vi "Read Loop.vi"(7 "Enum - Menu":enum16{"INIT", "READ", "RE-INIT", "CLOSE"}(ring), 8 "error in (no error)":errorcluster) -> (0 "error out":errorcluster, 1 "Isolated Gain":u32, 2 "DAQ Status":u32, 3 "Downlink Packet":T1)   [LabVIEW 2025]
panel:
  out "error out 2":errorcluster
  out "connection ID":refnum<k16>
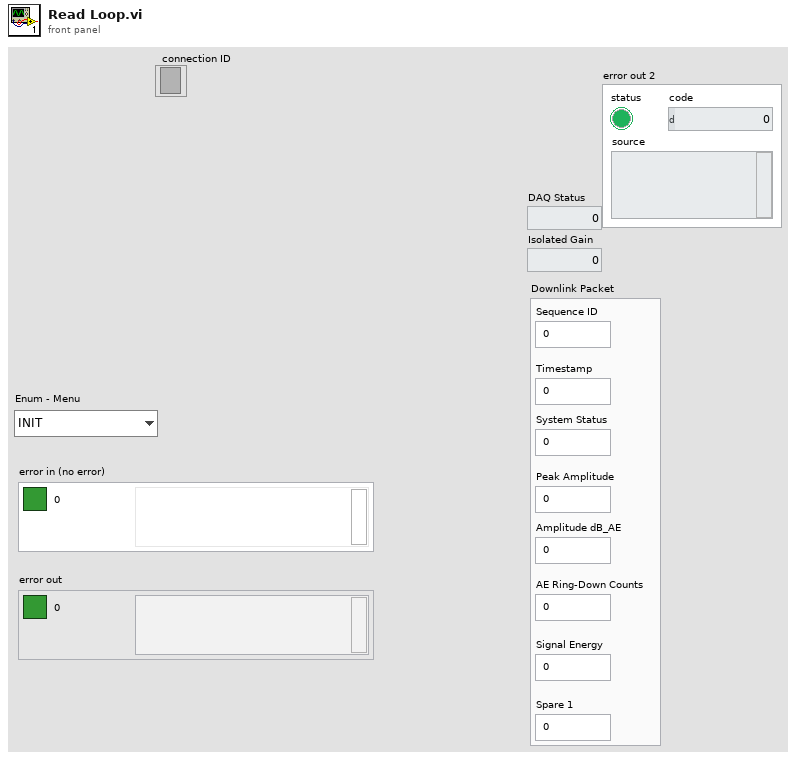
[diagram p1: front panel]
types:
  T1 = cluster{"Sequence ID":u32, "Timestamp":u32, "System Status":u32, "Peak Amplitude":u32, "Amplitude dB_AE":u32, "AE Ring-Down Counts":u32, "Signal Energy":u32, "Spare 1":u32}
  T2 = enum16{"big-endian, network order", "native, host order", "little-endian"}
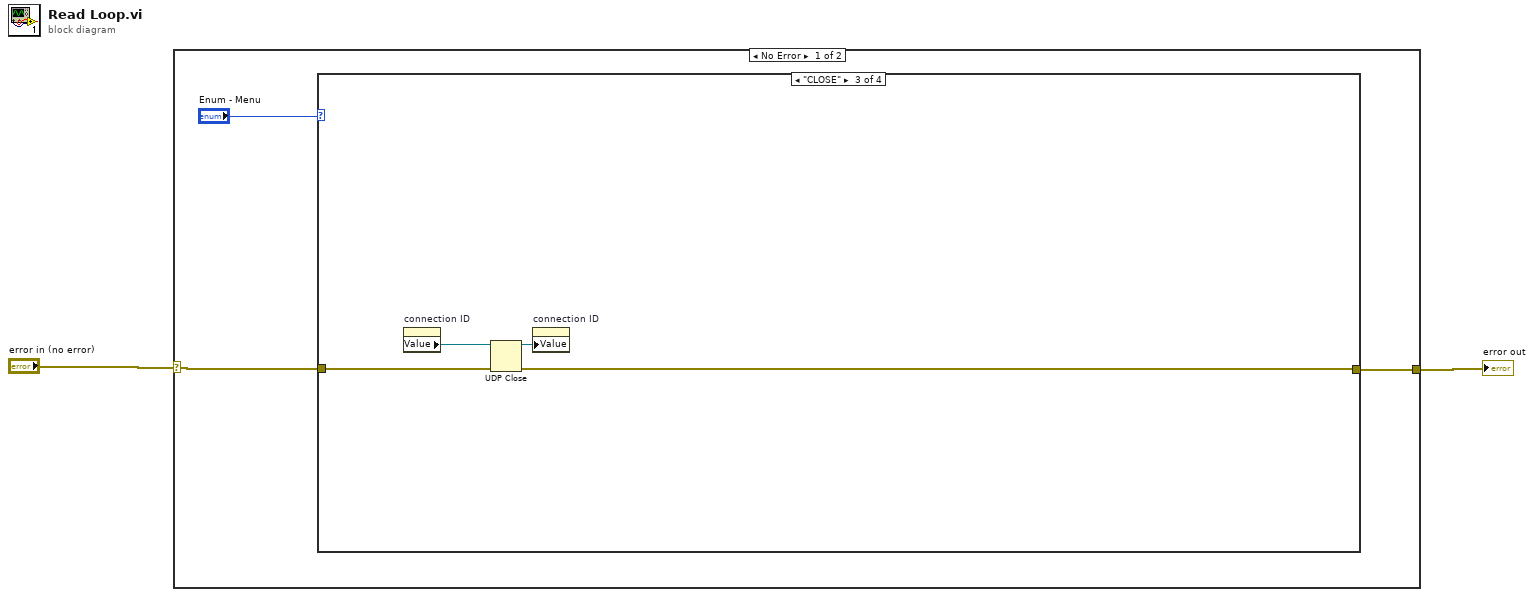
[diagram p0: block diagram]
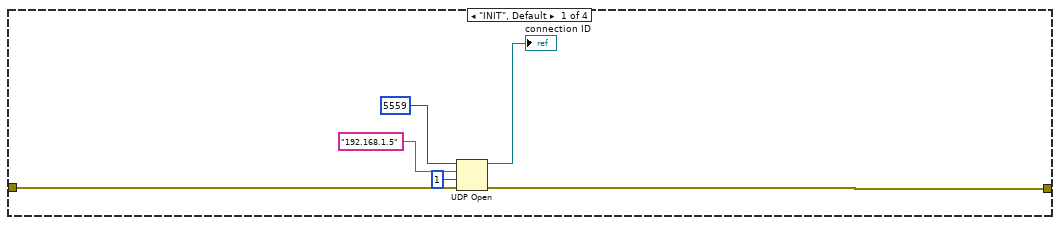
[diagram p2: hidden frame]
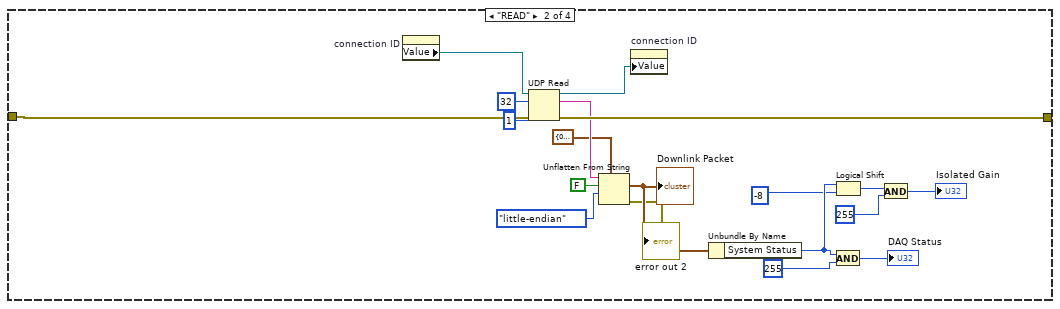
[diagram p3: hidden frame]
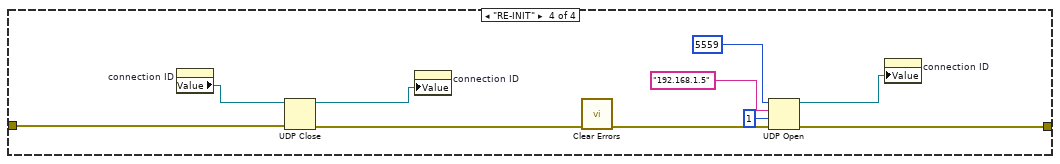
[diagram p4: hidden frame]
diagram:
  n1 = case shown="No Error" "error in (no error)" {
    selector: "error in (no error)" -> [w4 _]
    tunnel: [w3 _] -> w1
    frame No Error {
      n2 = case shown="\"CLOSE\"" "Enum - Menu" {
        tunnel: w4 -> [w10 w30 w32 w44]
        tunnel: [w9 w29 w31 w38] -> w3
        frame "INIT", Default {
          n3 = UDP Open(8:w10, 9:1 ("timeout ms (25000)"), 10:"192.168.1.5" ("service name"), 11:u16 5559 ("port")) -> (port=→"connection ID":refnum<k16>, 0:w9:errorcluster)  [unwired: 1 in, 1 out]
        }
        frame "READ" {
          n4 = property on="connection ID" class="Ref (strict)"() -> ("Value"=w27:refnum<k16>)  [unwired: 2 in, 2 out]
          n5 = UDP Read(connection ID=w27, max size (548)=32, timeout ms (25000)=1, 8:w30) -> (data out=w22:string, error out=w29:errorcluster, 3:w28:refnum<k16>)  [unwired: 2 out]
          n6 = Unflatten From String(type=T1 {"Sequence ID"=0, "Timestamp"=0, "System Status"=0, "Peak Amplitude"=0, "Amplitude dB_AE"=0, "AE Ring-Down Counts"=0, "Signal Energy"=0, "Spare 1"=0} ("Downlink Packet"), binary string=w22, data includes array or string size? (T)=FALSE ("prepend array or string size? (T)"), byte order (0:big-endian, network order)=T2."little-endian") -> (value=w20:T1, error out=→"error out 2":errorcluster)  [unwired: 1 in, 1 out]
          "Downlink Packet" <- w20
          n7 = property on="connection ID" class="Ref (strict)"("Value"=w28) -> ()  [unwired: 2 in, 2 out]
          n8 = Unbundle By Name(w20) -> ("System Status"=w17:u32)
          n9 = Logical Shift(y=w17, x=-8) -> (x << y=w15:i32)
          n10 = And(x=w17, y=u32 255) -> (x .and. y?=→"DAQ Status":u32)
          n11 = And(x=w15, y=u32 255) -> (x .and. y?=→"Isolated Gain":u32)
        }
        frame "CLOSE" {
          n12 = property on="connection ID" class="Ref (strict)"() -> ("Value"=w34:refnum<k16>)  [unwired: 2 in, 2 out]
          n13 = UDP Close(connection ID=w34, 8:w32) -> (connection ID out=w33:refnum<k16>, error out=w31:errorcluster)
          n14 = property on="connection ID" class="Ref (strict)"("Value"=w33) -> ()  [unwired: 2 in, 2 out]
        }
        frame "RE-INIT" {
          n15 = property on="connection ID" class="Ref (strict)"() -> ("Value"=w43:refnum<k16>)  [unwired: 2 in, 2 out]
          n16 = UDP Close(connection ID=w43, 8:w44) -> (connection ID out=w42:refnum<k16>, error out=w39:errorcluster)
          n17 = property on="connection ID" class="Ref (strict)"("Value"=w42) -> ()  [unwired: 2 in, 2 out]
          n18 = call <vilib>:"Clear Errors.vi"("error in (no error)"=w39) -> ("error out"=w36:errorcluster)  [unwired: 5 in, 1 out]
          n19 = UDP Open(8:w36, 9:1 ("timeout ms (25000)"), 10:"192.168.1.5" ("service name"), 11:u16 5559 ("port")) -> (port=w37:refnum<k16>, 0:w38:errorcluster)  [unwired: 1 in, 1 out]
          n20 = property on="connection ID" class="Ref (strict)"("Value"=w37) -> ()  [unwired: 2 in, 2 out]
        }
      }
    }
    frame Error {
    }
  }
  "error out" <- w1
